vi "LDA_interp&spectra.vi"() -> (5 "Plug in titles":string[](array[string]), 7 "Plug in values":string[](array[string]))   [LabVIEW 2010]
uses:
  Globals/LDA_meas_global_1.vi
  Globals/Plug_in_data_global.vi
  Globals/Meas_global.vi
  <vilib>/measure/maresamp.llb/Resample Pair of Arrays (single shot).vi
  <vilib>/Analysis/4window.llb/Hamming Window (DBL).vi
  <vilib>/measure/NI_MAPro.lvlib
  <vilib>/Analysis/NI_AALPro.lvlib
panel:
  in  "Desired Component":i32(ring) items=["LDA (U)", "LDA (W)"]
  out "Valid Blocks":i32
  out "Resampl.freq.(Hz)":dbl
  out "Length of block (s)":dbl
  out "Min length of processable block (s)":dbl
  out "Max length of processable block (s)":dbl
  in  "Points per block":dbl
  in  "Av.data rate(Hz)":dbl
  out "Frequency Spectrum":cluster{dbl, dbl, dbl[]}(graph)
  out "No Of Samples":i32
  # "You must have just these two indicators on the connector pane of the vi"
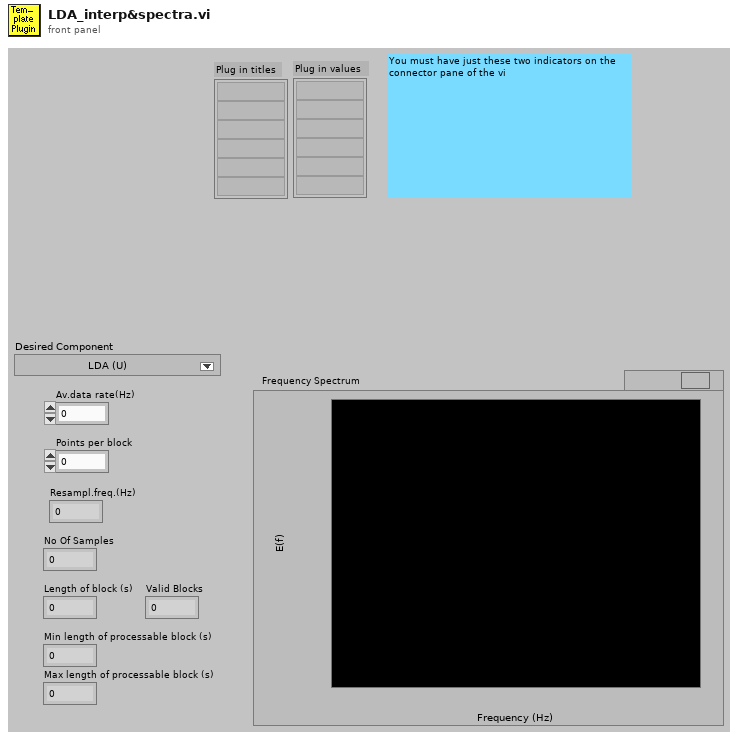
[diagram p1: front panel]
types:
  T1 = typedef "Analysis_info_cluster.ctl" = cluster{"Colour":u32, "Inst type":T2, "Inst name":string, "Symbol":string, "Code name":string, "Extra Info":string, "Inst Array":T3, "Index":i32, "Voltage Index":i32, "Extra Titles":string[], "Extra Values":string[]}
  T2 = typedef "Inst_type.ctl" = enum16{"Propeller anemometer", "Raw voltage", "Pressure Transducer", "Pitot-static tube", "Preston tube", "Hot wire", "Cross wire 1", "Cross wire 2", "Generic Linear", "Generic Polynomial", "Generic BackPoly", "Fast FID", "Thermocouple", "Cold wire", "Pulsed Wire", "LDA Vel", "LDA Tran time", "LDA Arr time"}
  T3 = typedef "Instrument_Array.ctl" = enum16{"PWA", "LDA", "Analogue"}
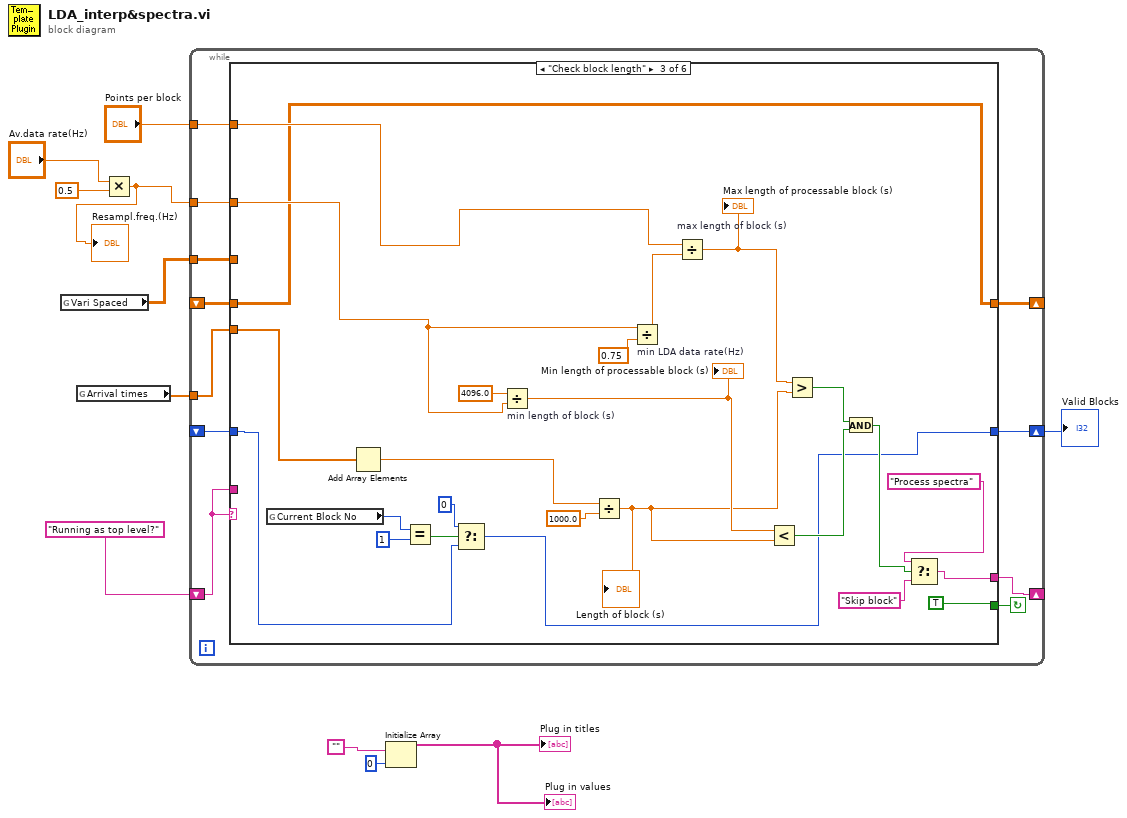
[diagram p0: block diagram]
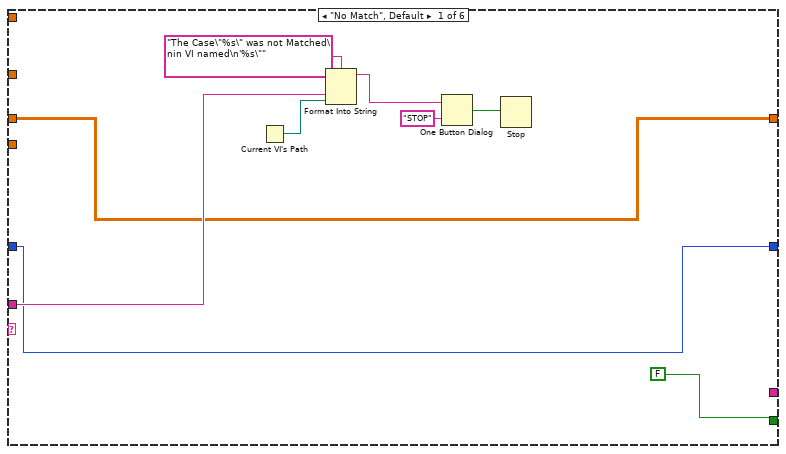
[diagram p2: hidden frame]
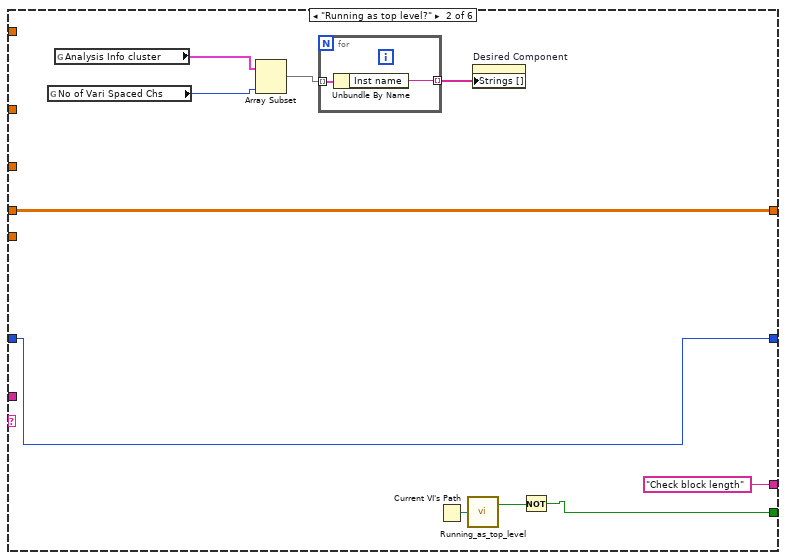
[diagram p3: hidden frame]
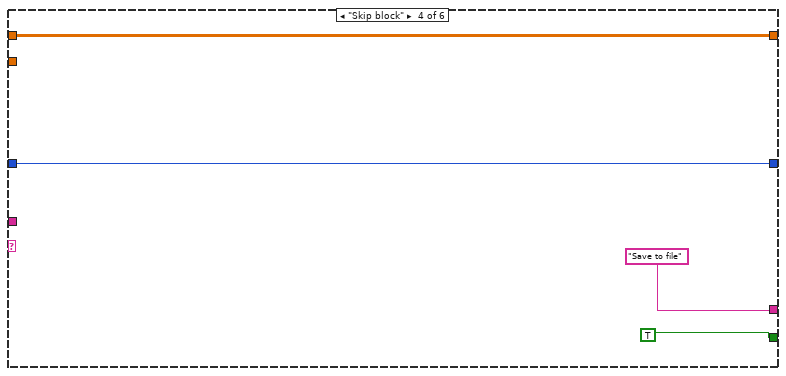
[diagram p4: hidden frame]
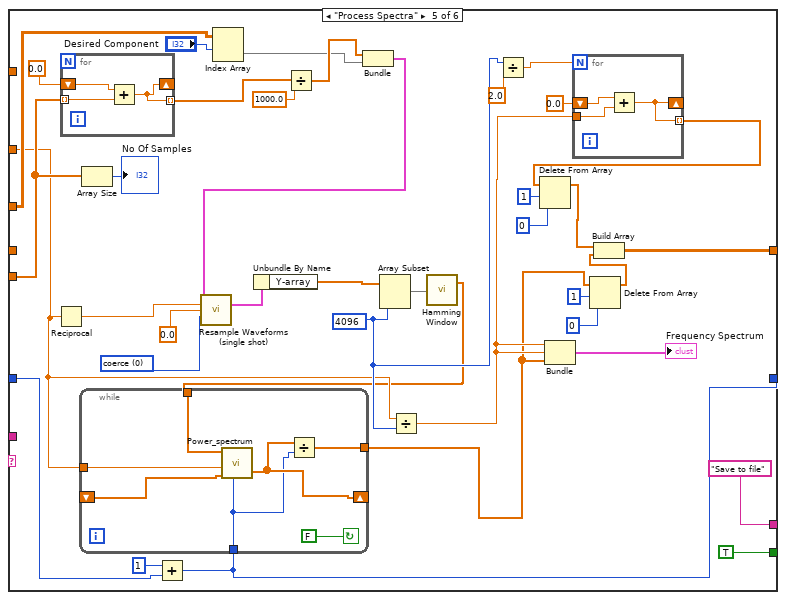
[diagram p5: hidden frame]
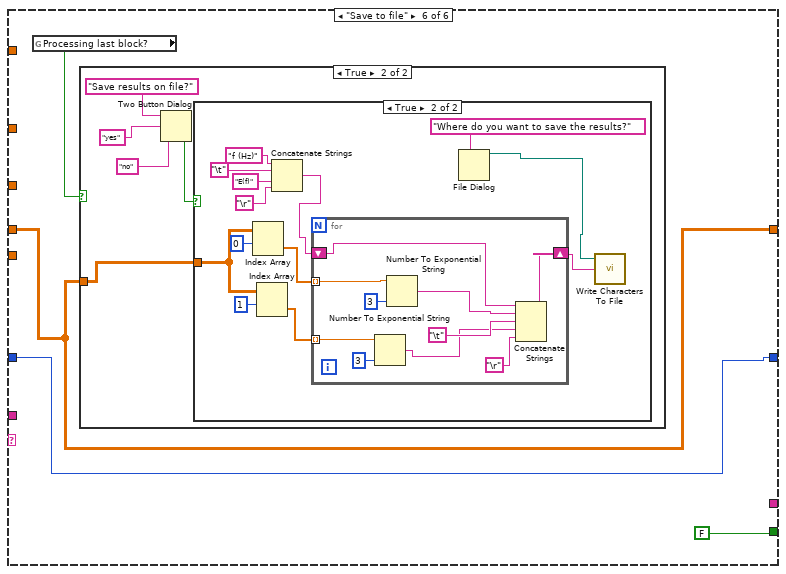
[diagram p6: hidden frame]
diagram:
  n1 = global read "Plug_in_data_global.vi" "Vari Spaced"() -> (w10:dbl[][])
  n2 = global read "LDA_meas_global_1.vi" "Arrival times"() -> (w9:dbl[])
  n3 = Multiply(x="Av.data rate(Hz)", y=0.5) -> (x*y=w2:dbl)
  "Resampl.freq.(Hz)" <- w2
  n4 = while {
    shift-left: "Running as top level?" -> [w22]
    shift-right: [w18] -> _
    tunnel: w10 -> [w21]
    tunnel: w9 -> [w20]
    tunnel: "Points per block" -> [w19]
    shift-right: [w12] -> w1
    shift-left: _ -> [w16]
    shift-right: [w15] -> _
    shift-left: _ -> [w14]
    tunnel: w2 -> [w13]
    stop <- w17 continue-if-true
    n5 = case shown="\"Check block length\"" w22 {
      tunnel: [_ "Check block length" w55 "Save to file" "Save to file" _] -> w18
      tunnel: w22 -> [w27 _ _ _ _ _]
      tunnel: w21 -> [_ _ _ _ w92 _]
      tunnel: w20 -> [_ _ w58 _ w93 _]
      tunnel: w19 -> [_ _ w65 _ _ _]
      tunnel: [FALSE w37 TRUE TRUE TRUE FALSE] -> w17
      tunnel: w16 -> [w24 w41 w47 w70 w85 w125]
      tunnel: [w23 w40 w44 w69 w87 w124] -> w15
      tunnel: w14 -> [w23 w40 w44 w69 _ w124]
      tunnel: w13 -> [_ _ w51 _ w86 _]
      tunnel: [w24 w41 w46 w70 w84 w125] -> w12
      frame "No Match", Default {
        n6 = Current VI's Path() -> (path=w26:path)
        n7 = Format Into String(format string="The Case\"%s\" was not Matched\nin VI named\n'%s\"" ("Format String"), w27, w26) -> (resulting string=w30:string)  [unwired: 2 in, 1 out]
        n8 = One Button Dialog(message=w30, button name ("OK")="STOP") -> (true=w28:bool)
        n9 = Stop(stop? (T)=w28) -> ()
      }
      frame "Running as top level?" {
        n10 = global read "Meas_global.vi" "No of Vari Spaced Chs"() -> (w34:i32)
        n11 = global read "Meas_global.vi" "Analysis Info cluster"() -> (w35:T1[])
        n12 = Array Subset(array=w35, length=w34) -> (w33:T1[])  [unwired: 1 in]
        n13 = for {
          tunnel: w33 -> [w43] mode=indexing
          tunnel: [w42] -> w32 mode=indexing
          n14 = Unbundle By Name(w43) -> ("Inst name"=w42:string)
        }
        n15 = Current VI's Path() -> (path=w39:path)
        n16 = call "Running_as_top_level.vi"("Vi path name"=w39) -> ("Top Level"=w38:bool)  [unwired: 1 out]
        n17 = property on="Desired Component" class="Ring (strict)"("Strings []"=w32) -> ()  [unwired: 2 in, 2 out]
        n18 = Not(x=w38) -> (.not. x?=w37:bool)
      }
      frame "Check block length" {
        n19 = global read "Meas_global.vi" "Current Block No"() -> (w50:i32)
        n20 = Add Array Elements(numeric array=w58) -> (sum=w57:dbl)
        n21 = Equal?(x=w50, y=1) -> (x = y?=w48:bool)
        n22 = Select(t=0, s=w48, f=w47) -> (s? t:f=w46:i32)
        n23 = Divide "min length of block (s)"(x=4096.0, y=w51) -> (x/y=w62:dbl)
        "Min length of processable block (s)" <- w62
        n24 = Divide(x=w57, y=1000.0) -> (x/y=w52:dbl)
        "Length of block (s)" <- w52
        n25 = Divide "min LDA data rate(Hz)"(x=w51, y=0.75) -> (x/y=w66:dbl)
        n26 = Divide "max length of block (s)"(x=w65, y=w66) -> (x/y=w63:dbl)
        "Max length of processable block (s)" <- w63
        n27 = Less?(x=w62, y=w52) -> (x < y?=w60:bool)
        n28 = Greater?(x=w63, y=w52) -> (0:w61:bool)
        n29 = And(x=w61, y=w60) -> (x .and. y?=w59:bool)
        n30 = Select(t="Process spectra", s=w59, f="Skip block") -> (s? t:f=w55:string)
      }
      frame "Skip block" {
      }
      frame "Process Spectra" {
        w95 = 4096 ("length")
        w107 = u16 0 items=["coerce", "linear", "spline", "FIR filter"] ("interpolation mode")
        (unwired) FALSE
        n31 = Reciprocal(x=w86) -> (1/x=w101:dbl)
        n32 = for {
          shift-right: [w121] -> _
          shift-left: 0.0 -> [w123]
          tunnel: w93 -> [w122] mode=indexing
          tunnel: [w121] -> w91 mode=indexing
          n33 = Add(x=w123, y=w122) -> (x+y=w121:dbl)
        }
        n34 = Array Size(array=w93) -> (size(s)=→"No Of Samples":i32)
        n35 = Add(x=1, y=w85) -> (x+y=w84:i32)
        n36 = Index Array(array=w92, index (row)="Desired Component") -> (element=w104:dbl[])  [unwired: 1 in]
        n37 = Divide(x=w91, y=1000.0) -> (x/y=w105:dbl[])
        n38 = Bundle(w105, "Vari Spaced"=w104) -> (w103:cluster{dbl[], "Vari Spaced":dbl[]})  [unwired: 1 in]
        n39 = call-poly <vilib>:"Resample Waveforms (single shot).vi"("XY-data in"=w103, "dt"=w101, "t0"=0.0, "interpolation mode"=w107) -> ("XY-data out"=w99:cluster{"X-array":dbl[], "Y-array":dbl[]})  [unwired: 7 in, 4 out]
        n40 = Unbundle By Name(w99) -> ("Y-array"=w100:dbl[])
        n41 = Array Subset(array=w100, length=w95) -> (w83:dbl[])  [unwired: 1 in]
        n42 = Divide(x=w86, y=w95) -> (x/y=w97:dbl)
        n43 = call-poly <vilib>:"Hamming Window.vi"("X"=w83) -> ("Windowed X"=w82:dbl[])  [unwired: 1 out]
        n44 = while {
          tunnel: w84 -> [w116]
          tunnel: w86 -> [w120]
          shift-right: [w117] -> _
          shift-left: _ -> [w119]
          tunnel: w82 -> [w118]
          tunnel: [w114] -> w74
          stop <- FALSE continue-if-true
          n45 = call "Power_spectrum.vi"("U"=w118, "Sampling frequency"=w120, "Spectrum input array"=w119, "Block No"=w116) -> ("Spectrum output array"=w117:dbl[])  [unwired: 2 in]
          n46 = Divide(x=w117, y=w116) -> (x/y=w114:dbl[])
        }
        n47 = Divide(x=w95, y=2.0) -> (x/y=w94:dbl)
        n48 = Bundle(w97, w97, w74) -> (→"Frequency Spectrum":cluster{dbl, dbl, dbl[]})  [unwired: 1 in]
        n49 = for {
          N: w94 -> [_]
          shift-right: [w112] -> _
          shift-left: 0.0 -> [w113]
          tunnel: [w112] -> w78 mode=indexing
          tunnel: w97 -> [w111]
          n50 = Add(x=w113, y=w111) -> (x+y=w112:dbl)
        }
        n51 = Delete From Array(array=w78, length=1, index=0) -> (array with subset deleted=w79:dbl[])  [unwired: 1 out]
        n52 = Delete From Array(array=w74, length=1, index=0) -> (array with subset deleted=w75:dbl[])  [unwired: 1 out]
        n53 = Build Array(w79, w75) -> (w87:dbl[][])
      }
      frame "Save to file" {
        n54 = global read "Meas_global.vi" "Processing last block?"() -> (w127:bool)
        n55 = case shown="True" w127 {
          tunnel: w124 -> [_ w132]
          frame False {
          }
          frame True {
            n56 = Two Button Dialog(message="Save results on file?", 1:"no", 2:"yes") -> (T button?=w128:bool)
            n57 = case shown="True" w128 {
              tunnel: w132 -> [_ w143]
              frame False {
              }
              frame True {
                n58 = Index Array(array=w143, index (row)=0) -> (element=w140:dbl[])  [unwired: 1 in]
                n59 = Index Array(array=w143, index (row)=1) -> (element=w138:dbl[])  [unwired: 1 in]
                n60 = Concatenate Strings("f (Hz)", "\t", "E(f)", "\r") -> (w133:string)
                n61 = for {
                  shift-right: [w148] -> w141
                  shift-left: w133 -> [w149]
                  tunnel: w140 -> [w147] mode=indexing
                  tunnel: w138 -> [w146] mode=indexing
                  n62 = Number To Exponential String(number=w146, precision (6)=i16 3) -> (E-format string=w151:string)  [unwired: 2 in]
                  n63 = Number To Exponential String(number=w147, precision (6)=i16 3) -> (E-format string=w154:string)  [unwired: 2 in]
                  n64 = Concatenate Strings(w149, w154, "\t", w151, "\r") -> (w148:string)
                }
                n65 = File Dialog(7:"Where do you want to save the results?" ("prompt")) -> (3:w139:path)  [unwired: 6 in, 3 out]
                n66 = call <vilib>:"Write Characters To File.vi"("character string"=w141, "file path (dialog if empty)"=w139) -> ()  [unwired: 3 in, 1 out]
              }
            }
          }
        }
      }
    }
  }
  "Valid Blocks" <- w1
  n67 = Initialize Array("", 0) -> (→"Plug in values" →"Plug in titles":string[])
